vi "StartWindowDrag.vi"(8 "error in (no error)":errorcluster, 11 "VI Ref (calling VI)":refnum<vi>) -> (0 "error out":errorcluster, 3 "dup VI Ref":refnum<vi>)   [LabVIEW 2025, in "WindowFrame.lvlib" / "WindowFrame.lvclass"]
uses:
  WindowFrame.lvclass
  user32.dll
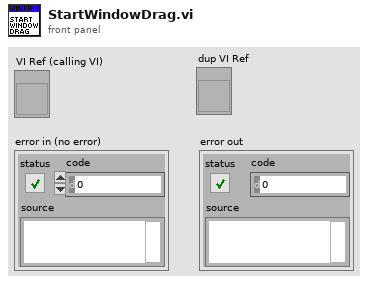
[diagram p1: front panel]
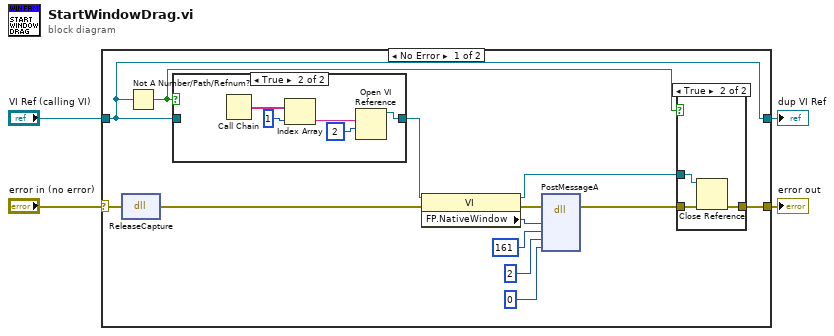
[diagram p0: block diagram]
diagram:
  n1 = case shown="No Error" "error in (no error)" {
    selector: "error in (no error)" -> [w17 w29]
    tunnel: "VI Ref (calling VI)" -> [w5 w28]
    tunnel: [w6 w29] -> w4
    tunnel: [w5 w28] -> w1
    frame No Error {
      n2 = dll-call lib="user32.dll" fn="ReleaseCapture"(error in=w17) -> (error out=w16:errorcluster)  [unwired: 3 in, 1 out]
      n3 = Not A Number/Path/Refnum?(number/path/refnum=w5) -> (NaN/Path/Refnum?=w10:bool)
      n4 = case shown="True" w10 {
        tunnel: [w22 w23] -> w9
        tunnel: w5 -> [w22 _]
        frame False {
        }
        frame True {
          n5 = Call Chain() -> (call chain=w27:string[])
          n6 = Index Array(array=w27, index=1 ("Index")) -> (element=w25:string)
          n7 = Open VI Reference(vi path=w25, options=2) -> (vi reference=w23:refnum<vi>)  [unwired: 4 in, 1 out]
        }
      }
      n8 = property class="VI"(reference=w9, error in=w16) -> (reference out=w8:refnum<vi>, error out=w15:errorcluster, "FP.NativeWindow"=w14:u64)
      n9 = dll-call lib="user32.dll" fn="PostMessageA"(error in=w15, "hWnd"=w14, "Msg"=161, "wParam"=2, "lParam"=0) -> (error out=w7:errorcluster)  [unwired: 7 in, 1 out]
      n10 = case shown="True" w10 {
        tunnel: w8 -> [_ w21]
        tunnel: w7 -> [w18 w20]
        tunnel: [w18 w19] -> w6
        frame False {
        }
        frame True {
          n11 = Close Reference(reference=w21, error in (no error)=w20) -> (error out=w19:errorcluster)
        }
      }
    }
    frame Error {
    }
  }
  "error out" <- w4
  "dup VI Ref" <- w1
